vi "NGTS_DAQmx_Initialize_AO.vi"(8 "error in":errorcluster, 10 "Channels Properties Table":string[][](array[string])) -> (0 "error out":errorcluster, 2 "AO Task Array Out":refnum<k21>[](array[refnum]))   [LabVIEW 2018]
doc: "Creates tasks based on \"Number_of_SCXI_Chassis\" entry in the AO_Configuration section of the Config_INI file. (Defaulted to 2 at this time). It then populates the tasks with Channels created from rows in the Channel Properties Table. The Tasks are optionally saved in MAX. If not, the the Auto Cleanup of Tasks is TRUE and LabVIEW will automatically clean up Tasks of completion of execution of the application.\n\n2007-11 Mike Ashe\nmichael.ashe@imaginatics.net\nCell: 860-961-0876"
uses:
  <vilib>/DAQmx/create/channels.llb/DAQmx Create Channel (AO-Voltage-Basic).vi
  <vilib>/DAQmx/create/channels.llb/DAQmx Create Channel (AO-Current-Basic).vi
panel:
  in  "Save Virtual Channels":bool
  in  "Author":string="Mike Ashe"
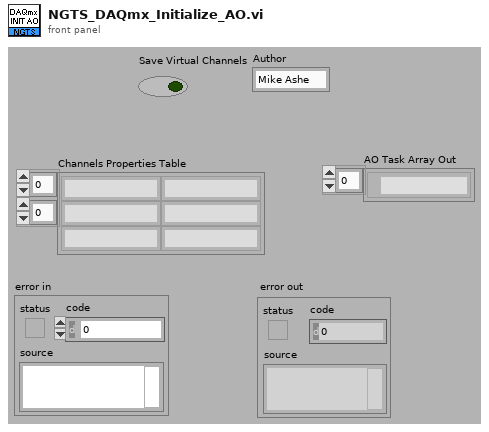
[diagram p1: front panel]
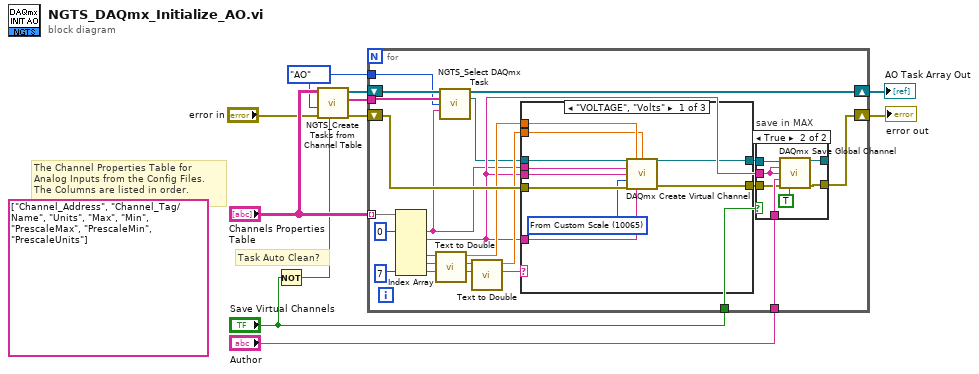
[diagram p0: block diagram]
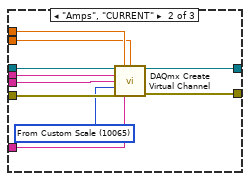
[diagram p2: hidden frame]
diagram:
  w2 = enum16{"AI", "AO", "DI", "DO"}."AO" ("Type of IO")
  (unwired) string[] ["Channel_Address", "Channel_Tag/Name", "Units", "Max", "Min", "PrescaleMax", "PrescaleMin", "PrescaleUnits"]
  # "Task Auto Clean?"
  # "The Channel Properties Table for\nAnalog Inputs from the Config Files.\nThe Columns are listed in order."
  n1 = Not(x="Save Virtual Channels") -> (.not. x?=w4:bool)
  n2 = call "NGTS_Create Tasks from Channel Table.vi"("Task Auto Cleanup?"=w4, "error in"="error in", "Type of IO"=w2, "Channels Properties Table"="Channels Properties Table") -> ("error out"=w8:errorcluster, "List of Devices"=w3:string[], "DAQmx Task Array Out"=w6:refnum<k21>[])  [unwired: 5 in]
  n3 = for {
    shift-right: [w12] -> w10
    shift-left: w6 -> [w17]
    tunnel: "Author" -> [w32]
    tunnel: "Save Virtual Channels" -> [w31]
    tunnel: "Channels Properties Table" -> [w30] mode=indexing
    shift-right: [w26] -> w9
    shift-left: w8 -> [w24]
    tunnel: w3 -> [w14]
    tunnel: w2 -> [w13]
    n4 = Index Array(array=w30, index #1=0 ("index"), index #6=7 ("index")) -> (element #1=w15:string, element #2=w18:string, element #4=w29:string, element #5=w28:string, element #6=w19:string)  [unwired: 4 in, 1 out]
    n5 = call "Text to Double.vi"("string"=w29) -> ("number"=w23:dbl)  [unwired: 10 in]
    n6 = call "NGTS_Select DAQmx Task.vi"("DAQmx Tasks In"=w17, "List of Devices"=w14, "Type of IO"=w13, "Channel Address"=w15) -> ("DAQmx Tasks Out"=w12:refnum<k21>[], "DAQmx Task Selected Out"=w16:refnum<k21>)  [unwired: 9 in, 1 out]
    n7 = call "Text to Double.vi"("string"=w28) -> ("number"=w22:dbl)  [unwired: 10 in]
    n8 = case shown="\"VOLTAGE\", \"Volts\"" w19 {
      tunnel: w16 -> [w42 w52 w54]
      tunnel: w15 -> [w38 w51 _]
      tunnel: w22 -> [w33 w43 _]
      tunnel: w23 -> [w34 w44 _]
      tunnel: [w40 w50 w54] -> w21
      tunnel: [w39 w49 w53] -> w25
      tunnel: w18 -> [w37 w48 _]
      tunnel: w24 -> [w41 w47 w53]
      tunnel: w18 -> [w35 w45 _]
      frame "VOLTAGE", "Volts" {
        w36 = 10065 items=["Volts"=10348, "From Custom Scale"=10065] ("units")
        n9 = call-poly <vilib>:"DAQmx Create Virtual Channel.vi"("task in"=w42, "maximum value"=w34, "minimum value"=w33, "physical channels"=w38, "name to assign"=w37, "units"=w36, "error in"=w41, "custom scale name"=w35) -> ("task out"=w40:refnum<k21>, "error out"=w39:errorcluster)  [unwired: 6 in]
      }
      frame "Amps", "CURRENT" {
        w46 = 10065 items=["Amps"=10342, "From Custom Scale"=10065] ("units")
        n10 = call-poly <vilib>:"DAQmx Create Virtual Channel.vi"("task in"=w52, "maximum value"=w44, "minimum value"=w43, "physical channels"=w51, "name to assign"=w48, "units"=w46, "error in"=w47, "custom scale name"=w45) -> ("task out"=w50:refnum<k21>, "error out"=w49:errorcluster)  [unwired: 6 in]
      }
      frame Default {
      }
    }
    n11 = case "save in MAX" shown="True" w31 {
      tunnel: [w56 w63] -> _
      tunnel: w18 -> [_ w60]
      tunnel: w32 -> [_ w62]
      tunnel: [w55 w61] -> w26
      tunnel: w21 -> [w56 w59]
      tunnel: w25 -> [w55 w58]
      frame False {
      }
      frame True {
        n12 = call <vilib>:"DAQmx Save Global Channel.vi"("task/channels in"=w59, "channel name"=w60, "save as"=w60, "author"=w62, "error in"=w58, "overwrite existing channel?"=TRUE) -> ("task out"=w63:refnum<k21>, "error out"=w61:errorcluster)  [unwired: 8 in]
      }
    }
  }
  "AO Task Array Out" <- w10
  "error out" <- w9
